vi "Error Function.vi"(1 "Names":string[](array[string])=["Bc", "y", "mag", "theta", "v0", "v1", "v2", "g0", "width"], 2 "Array":dbl[](array[numeric])=[7.0, 0.61, 0.5, 1.522, 0.11, 0.36, 0.5, 0.24, 0.055, 1.0] format="%_4g") -> (0 "Error":dbl=6.318493677348696)   [LabVIEW 2016]
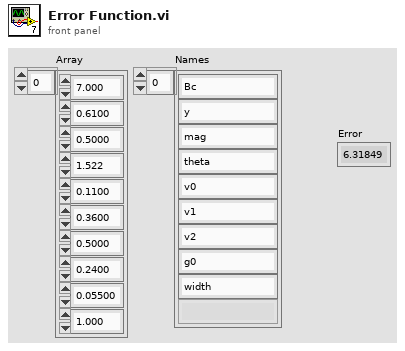
[diagram p1: front panel]
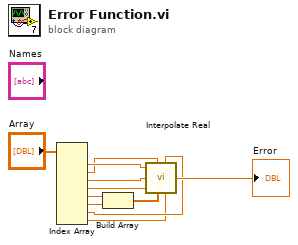
[diagram p0: block diagram]
diagram:
  n1 = Index Array(array="Array") -> (element #1=w11:dbl, element #2=w10:dbl, element #3=w9:dbl, element #4=w8:dbl, element #5=w7:dbl, element #6=w6:dbl, element #7=w2:dbl, element #8=w1:dbl)  [unwired: 8 in]
  n2 = Build Array(w7, w6) -> (w5:dbl[])
  n3 = call "Interpolate Real.vi"("Bc"=w11, "y"=w10, "Mag"=w9, "theta"=w8, "Initial"=w5, "g0"=w2, "width"=w1) -> ("sum"=→"Error":dbl)  [unwired: 2 in]
